vi "SubModule Read Data.vi"(8 "error in (no error)":errorcluster, 11 "Camera in":refnum<class "Camera.lvclass">) -> (0 "error out":errorcluster, 1 "Data":string[](array[string]), 3 "Camera out":refnum<class "Camera.lvclass">)   [LabVIEW 2021, in "Camera.lvclass"]
uses:
  Camera.lvclass
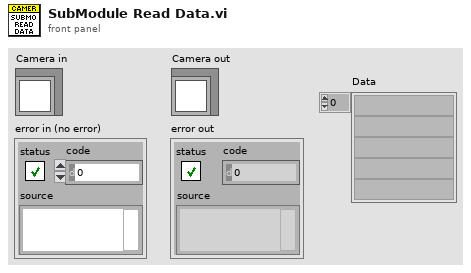
[diagram p1: front panel]
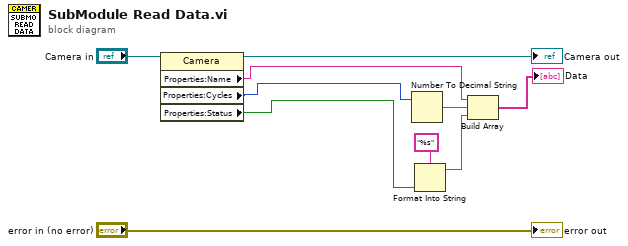
[diagram p0: block diagram]
diagram:
  n1 = property class="Camera"(reference="Camera in") -> (reference out=→"Camera out":refnum<class "Camera.lvclass">, "Properties:Name"=w1:string, "Properties:Cycles"=w2:i32, "Properties:Status"=w3:bool)  [unwired: 1 in, 1 out]
  n2 = Number To Decimal String(number=w2) -> (decimal integer string=w8:string)  [unwired: 1 in]
  n3 = Format Into String(format string="%s", w3) -> (resulting string=w7:string)  [unwired: 2 in, 1 out]
  n4 = Build Array(w1, w8, w7) -> (→"Data":string[])
  "error out" <- "error in (no error)"
